vi "Check for Done.vi"(0 "private data":T1={"GTX2_CHANNEL register map"=refnum, "instruction target"=refnum, "channel measure state"=enum."Uninitialized", "in DFE mode?"=FALSE, "prescale"=0, "rx internal data width"=enum."32 Bit", "active point"={"horizontal offset"=0, "vertical offset"=0}, "ut sign"=enum."Positive", "positive counts"={"sample count"=0, "error count"=0}, "negative counts"={"sample count"=0, "error count"=0}}, 5 "timeout (100 ms)":dbl=0.1, 11 "error in":errorcluster) -> (4 "private data out":T1={"GTX2_CHANNEL register map"=refnum, "instruction target"=refnum, "channel measure state"=enum."Uninitialized", "in DFE mode?"=FALSE, "prescale"=0, "rx internal data width"=enum."32 Bit", "active point"={"horizontal offset"=0, "vertical offset"=0}, "ut sign"=enum."Positive", "positive counts"={"sample count"=0, "error count"=0}, "negative counts"={"sample count"=0, "error count"=0}}, 6 "done?":bool, 8 "timed out?":bool, 10 "es control status":T7, 15 "error out":errorcluster)   [LabVIEW 2015, in "niHighSpeedSerial Eye Scan Single Point v1 Host.lvclass"]
doc: "Checks whether or not Eye Scan has completed sampling the point and moved into the DONE state.\n\n<B>Input Parameters</B>\n\n<B>private data</B> is the class private data input into the VI.\n\n<B>private data.GTX2_CHANNEL register map</B> is the GTX2 Channel register map to use.\n\n<B>private data.instruction target</B> is the instruction target to use when communicating with the FPGA.\n\n<B>private data.channel measure state</B> maintains the internal state of the Eye Scan Single Point class.\nenum values: Uninitialized,Initialized,Ready,Request,Wait,Read,Process,Finished\n\n<B>private data.in DFE mode?</B> is true if Eye Scan is configured for DFE Equalization Mode.\n\n<B>private data.prescale</B> controls scaling of the sample count in order to keep the sample count and error count within reasonable precision.\n\n<B>private data.receiver data width</B> is the data width (in bits) of the receiver lane.\nenum values: 16 Bit,20 Bit,32 Bit,40 Bit\n\n<B>private data.active point</B> is the point currently being sampled for errors using Eye Scan.\n\n<B>private data.active point.horizontal offset</B> is the horizontal offset of the active point.\n\n<B>private data.active point.vertical offset</B> is the vertical offset of the active point.\n\n<B>private data.ut sign</B> The untapped threshold sign (positive or negative) currently configured on the point being measured.\nPositive is used when in DFE or LPM Equalization Mode, while Negative is only used in DFE Equalization Mode.\n\n<B>private data.positive counts</B> contains the number of sample and error counts measured using the positive UT Sign.\n\n<B>private data.positive counts.sample count</B> is the positive sample count when using DFE mode, or the entire sample count when using LPM mode.\n\n<B>private data.positive counts.error count</B> is the positive error count when using DFE mode, or the entire error count when using LPM mode.\n\n<B>private data.negative counts</B> contains the number of sample and error counts measured using the negative UT Sign.\n\n<B>private data.negative counts.sample count</B> is the negative sample count when using DFE mode, or unused when using LPM mode.\n\n<B>private data.negative counts.error count</B> is the negative error count when using DFE mode, or unused when using LPM mode.\n\n<B>timeout (100 ms)</B> The amount of time (in seconds) before timing timing out.\nSpecifying '-1' prevents 'timed out' from ever returning true.\n\n<B>error in</B> describes error conditions that occur before this node runs. This input provides standard 'error in' functionality.\n\n<B>Output Parameters</B>\n\n<B>private data out</B> is the class private data output from the VI.\n\n<B>private data out.GTX2_CHANNEL register map</B> is the register map to use which represents the GTX2 Channel.\n\n<B>private data out.instruction target</B> is the instruction target to use when communicating with the FPGA.\n\n<B>private data out.channel measure state</B> maintains the internal state of the Eye Scan Single Point class.\nenum values: Uninitialized,Initialized,Ready,Request,Wait,Read,Process,Finished\n\n<B>private data out.in DFE mode?</B> is true if Eye Scan is configured for DFE Equalization Mode.\n\n<B>private data out.prescale</B> controls scaling of the sample count in order to keep the sample count and error count within reasonable precision.\n\n<B>private data out.receiver data width</B> is the data width (in bits) of the receiver lane.\nenum values: 16 Bit,20 Bit,32 Bit,40 Bit\n\n<B>private data out.active point</B> is the point currently being sampled for errors using Eye Scan.\n\n<B>private data out.active point.horizontal offset</B> is the horizontal offset of the active point.\n\n<B>private data out.active point.vertical offset</B> is the vertical offset of the active point.\n\n<B>private data out.ut sign</B> contains the number of sample and error counts measured using the positive UT Sign.\nenum values: Positive,Negative\n\n<B>private data out.positive counts</B> contains the number of sample and error counts measured using the positive UT Sign.\n\n<B>private data out.positive counts.sample count</B> is the positive sample count when using DFE mode, or the entire sample count when using LPM mode.\n\n<B>private data out.positive counts.error count</B> is the positive error count when using DFE mode, or the entire error count when using LPM mode.\n\n<B>private data out.negative counts</B> contains the number of sample and error counts measured using the negative UT Sign.\n\n<B>private data out.negative counts.sample count</B> is the negative sample count when using DFE mode, or the entire sample count when using LPM mode.\n\n<B>private data out.negative counts.error count</B> is the negative error count when using DFE mode, or the entire error count when using LPM mode.\n\n<B>done?</B> returns true if the Eye Scan algorithm has completed measuring all points.\n\n<B>timed out?</B> returns true if at least 'timeout' amount of time has passed.\n\n<B>es control status</B> is the current state of the Eye Scan engine on the target.\nenum values: Wait,Reset,End,Count,Read,Armed\n\n<B>error out</B> contains error information. This output provides standard 'error out' functionality."
uses:
  <instrlib>/niHighSpeedSerial/Eye Scan/v1/Host/Impl/Single Point/niHighSpeedSerial Eye Scan Single Point v1 Host.lvclass
  <instrlib>/niHighSpeedSerial/Register Maps/Xilinx/v1/Host/GTX2_CHANNEL v1 Host.llb/ESControlStatus.ctl
  <instrlib>/niHighSpeedSerial/Eye Scan/v1/Host/Impl/Single Point/Private/Private Data.ctl
  <instrlib>/niHighSpeedSerial/Register Maps/Xilinx/v1/Host/GTX2_CHANNEL v1 Host.llb/GTX2_CHANNEL Register Map.lvclass
  <instrlib>/_niInstr/Instruction Framework/v1/Host/Instruction Target/niInstr Instruction Target v1 Host.lvclass
  <instrlib>/niHighSpeedSerial/Eye Scan/v1/Host/Impl/Single Point/Private/Channel Measure State.ctl
  <instrlib>/niHighSpeedSerial/Eye Scan/v1/Host/Common/Public/Data Width.ctl
  <instrlib>/niHighSpeedSerial/Eye Scan/v1/Host/Common/Public/Point Offsets.ctl
  <instrlib>/niHighSpeedSerial/Register Maps/Xilinx/v1/Host/GTX2_CHANNEL v1 Host.llb/ESVertOffsetSign.ctl
  <instrlib>/niHighSpeedSerial/Eye Scan/v1/Host/Impl/Single Point/Private/Counts.ctl
  <instrlib>/niHighSpeedSerial/Register Maps/Xilinx/v1/Host/GTX2_CHANNEL v1 Host.llb/GTX2_CHANNEL Register Map.lvclass/GTX2_CHANNEL Register Map.ctl
  <instrlib>/niHighSpeedSerial/Register Maps/Xilinx/v1/Host/GTX2_CHANNEL v1 Host.llb/Read es_control_status.vi
  <instrlib>/niHighSpeedSerial/Register Maps/Xilinx/v1/Host/GTX2_CHANNEL v1 Host.llb/Decode Register to Address.vi
  <instrlib>/_niInstr/Instruction Framework/v1/Host/Instruction Target/Public/Context Read.vi
  <instrlib>/niHighSpeedSerial/Register Maps/Xilinx/v1/Host/GTX2_CHANNEL v1 Host.llb/GTX2_CHANNEL v1 Host.lvlib
  <instrlib>/niHighSpeedSerial/Eye Scan/v1/Host/Common/niHighSpeedSerial Eye Scan Common v1 Host.lvlib
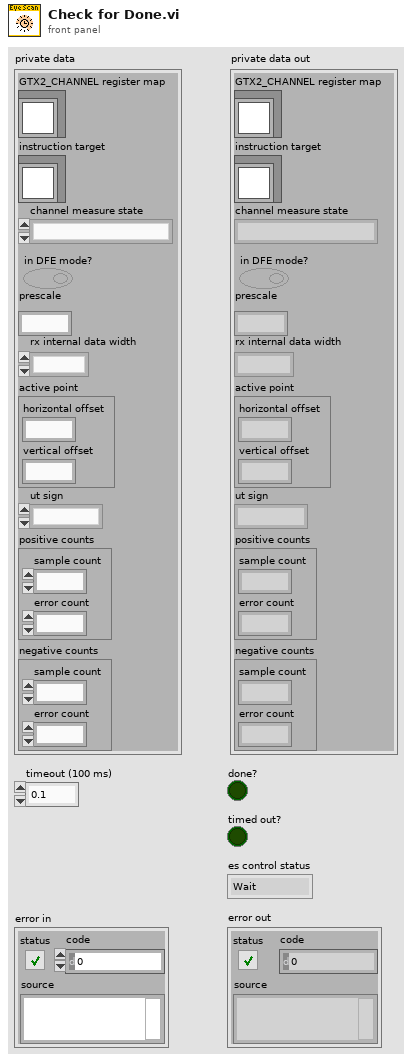
[diagram p1: front panel]
types:
  T1 = typedef "niHighSpeedSerial Eye Scan Single Point v1 Host.lvclass/Private Data.ctl" = cluster{"GTX2_CHANNEL register map":refnum<class "GTX2_CHANNEL Register Map.lvclass">, "instruction target":refnum<class "niInstr Instruction Target v1 Host.lvclass">, "channel measure state":T2, "in DFE mode?":bool, "prescale":u8, "rx internal data width":T3, "active point":T4, "ut sign":T5, "positive counts":T6, "negative counts":T6}
  T2 = typedef "niHighSpeedSerial Eye Scan Single Point v1 Host.lvclass/Channel Measure State.ctl" = enum16{"Uninitialized", "Initialized", "Ready", "Request", "Wait", "Read", "Process", "Finished"}
  T3 = typedef "niHighSpeedSerial Eye Scan Common v1 Host.lvlib/Data Width.ctl" = enum16{"16 Bit", "20 Bit", "32 Bit", "40 Bit"}
  T4 = typedef "niHighSpeedSerial Eye Scan Common v1 Host.lvlib/Point Offsets.ctl" = cluster{"horizontal offset":i16, "vertical offset":i8}
  T5 = typedef "GTX2_CHANNEL v1 Host.lvlib/ESVertOffsetSign.ctl" = enum8{"Positive", "Negative"}
  T6 = typedef "niHighSpeedSerial Eye Scan Single Point v1 Host.lvclass/Counts.ctl" = cluster{"sample count":u64, "error count":u16}
  T7 = typedef "GTX2_CHANNEL v1 Host.lvlib/ESControlStatus.ctl" = enum8{"Wait", "Reset", "End", "Count", "Read", "Armed"}
  T8 = typedef "GTX2_CHANNEL v1 Host.lvlib/es_control_status.ctl" = cluster{"done":bool, "es_control_status":T7, "RESERVED1":u16}
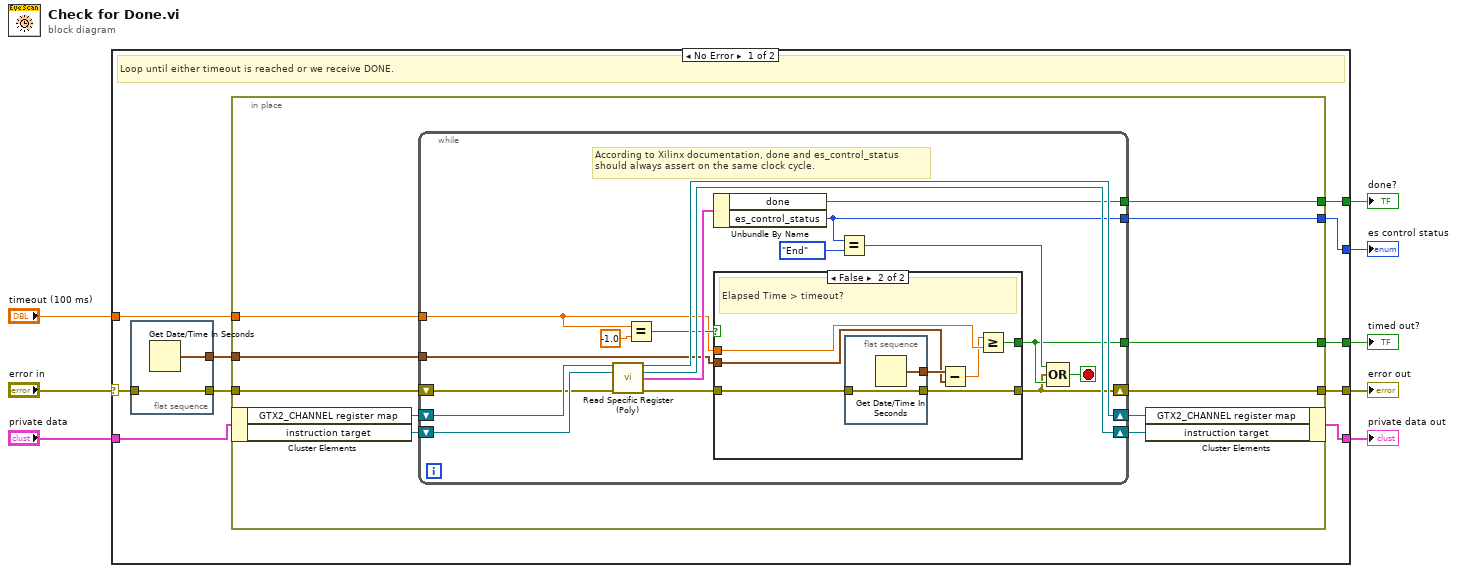
[diagram p0: block diagram]
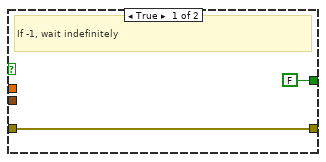
[diagram p2: hidden frame]
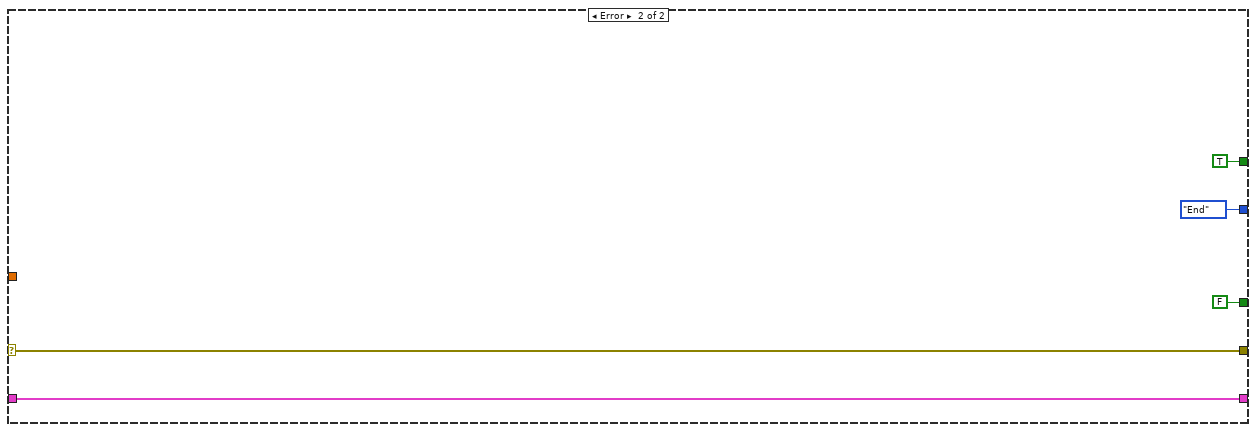
[diagram p3: hidden frame]
diagram:
  n1 = case shown="No Error" "error in" {
    selector: "error in" -> [w14 w65]
    tunnel: [w18 w65] -> w7
    tunnel: "timeout (100 ms)" -> [w17 _]
    tunnel: [w16 TRUE ("done")] -> w5
    tunnel: [w15 ESControlStatus."End" ("es_control_status")] -> w4
    tunnel: [w11 FALSE ("Time has Elapsed")] -> w3
    tunnel: "private data" -> [w10 w61]
    tunnel: [w9 w61] -> w1
    frame No Error {
      # "Loop until either timeout is reached or we receive DONE."
      n2 = flat-sequence {
        tunnel: w14 -> [w20]
        tunnel: [w20] -> w13
        tunnel: [w19] -> w12
        frame #0 {
          n3 = Get Date/Time In Seconds() -> (seconds since 1Jan1904=w19:timestamp)
        }
      }
      n4 = in-place {
        in-place-border: w13 -> [w31]
        in-place-border: [w25] -> w18
        in-place-border: w17 -> [w27]
        in-place-border: [w26] -> w16
        in-place-border: [w30] -> w15
        in-place-border: w12 -> [w29]
        in-place-border: [w28] -> w11
        n5 = in-place-cluster #1(w10) -> ("GTX2_CHANNEL register map"=w23:refnum<class "GTX2_CHANNEL Register Map.lvclass">, "instruction target"=w24:refnum<class "niInstr Instruction Target v1 Host.lvclass">)
        n6 = while {
          shift-right: [w32] -> w25
          shift-left: w31 -> [w34]
          shift-right: [w46] -> w22
          shift-left: w23 -> [w48]
          shift-right: [w45] -> w21
          shift-left: w24 -> [w47]
          tunnel: [w43] -> w26
          tunnel: [w39] -> w30
          tunnel: w29 -> [w37]
          tunnel: [w36] -> w28
          tunnel: w27 -> [w35]
          stop <- w49 stop-if-true
          # "According to Xilinx documentation, done and es_control_status\nshould always assert on the same clock cycle."
          n7 = call-poly <instrlib>:"Read Specific Register (Poly).vi"("gtx2_channel register map object in"=w48, "instruction target in"=w47, "error in"=w34) -> ("gtx2_channel register map object out"=w46:refnum<class "GTX2_CHANNEL Register Map.lvclass">, "instruction target out"=w45:refnum<class "niInstr Instruction Target v1 Host.lvclass">, "es_control_status"=w44:T8, "error out"=w33:errorcluster)  [unwired: 9 in]
          n8 = Equal?(x=w35, y=-1.0) -> (x = y?=w42:bool)
          n9 = Unbundle By Name(w44) -> ("done"=w43:bool, "es_control_status"=w39:T7)
          n10 = case shown="False" w42 {
            tunnel: [FALSE ("Time has Elapsed") w53] -> w36
            tunnel: w33 -> [w51 w58]
            tunnel: [w51 w57] -> w32
            tunnel: w35 -> [_ w56]
            tunnel: w37 -> [_ w54]
            frame True {
              # "If -1, wait indefinitely"
            }
            frame False {
              # "Elapsed Time > timeout?"
              n11 = flat-sequence {
                tunnel: [w60] -> w55
                tunnel: w58 -> [w59]
                tunnel: [w59] -> w57
                frame #0 {
                  n12 = Get Date/Time In Seconds() -> (seconds since 1Jan1904=w60:timestamp)
                }
              }
              n13 = Subtract(x=w55, y=w54) -> (x-y=w52:dbl)
              n14 = Greater Or Equal?(x=w52, y=w56) -> (x >= y?=w53:bool)
            }
          }
          n15 = Equal?(x=w39, y=ESControlStatus."End" ("es_control_status")) -> (x = y?=w40:bool)
          n16 = Compound Arithmetic op=OR(w40, w32, w36) -> (w49:bool)
        }
        n17 = in-place-cluster #1("GTX2_CHANNEL register map"=w22, "instruction target"=w21) -> (w9:T1)
      }
    }
    frame Error {
    }
  }
  "error out" <- w7
  "done?" <- w5
  "es control status" <- w4
  "timed out?" <- w3
  "private data out" <- w1
